vi "VisionDriver.vi"() -> (0 "horizontal":T2, 1 "vertical":T1)   [LabVIEW 2015]
uses:
  Robot Vision/horizontal.ctl
  Robot Vision/vertical.ctl
  Robot Vision/Robot Global Data.vi
panel:
  out "Distance (ft)":dbl
  out "Up":bool
  out "Down":bool
  out "Straight":bool
  out "Right":bool=TRUE
  out "Left":bool=TRUE
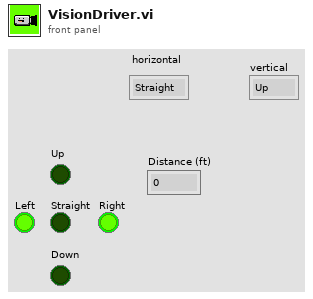
[diagram p1: front panel]
types:
  T1 = typedef "vertical.ctl" = enum16{"Up", "Down", "Straight"}
  T2 = typedef "horizontal.ctl" = enum16{"Straight", "Right", "Left"}
  T3 = cluster{"Distance (ft)":dbl, "Center":cluster{dbl, dbl}, "Normalized Rect":cluster{"Numeric":dbl, "Numeric 2":dbl, "Numeric 3":dbl, "Numeric 5":dbl}}[]
  T4 = cluster{"Distance (ft)":dbl, "Center":cluster{dbl, dbl}, "Normalized Rect":cluster{"Numeric":dbl, "Numeric 2":dbl, "Numeric 3":dbl, "Numeric 5":dbl}}
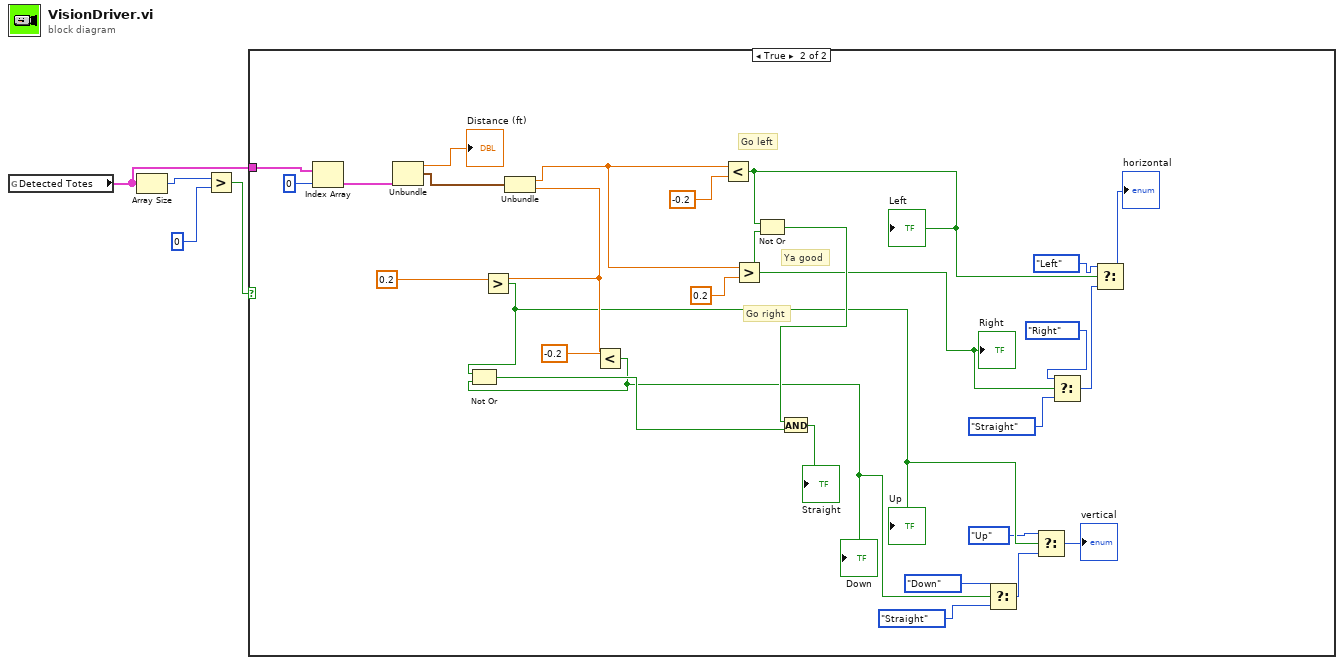
[diagram p0: block diagram]
diagram:
  n1 = global read "Robot Global Data.vi" "Detected Totes"() -> (w1:T3)
  n2 = Array Size(array=w1) -> (size(s)=w4:i32)
  n3 = Greater?(x=w4, y=0) -> (0:w2:bool)
  n4 = case shown="True" w2 {
    tunnel: w1 -> [_ w30]
    frame False {
    }
    frame True {
      # "Ya good"
      # "Go right"
      # "Go left"
      n5 = Index Array(array=w30, index=0) -> (element=w32:T4)
      n6 = Unbundle(w32) -> ("Distance (ft)"=→"Distance (ft)":dbl, "Center"=w29:cluster{dbl, dbl})  [unwired: 1 out]
      n7 = Unbundle(w29) -> (w28:dbl, w23:dbl)
      n8 = Greater?(x=w23, y=0.2 ("x")) -> (0:w11:bool)
      "Up" <- w11
      n9 = Less?(x=w23, y=-0.2 ("x")) -> (x < y?=w7:bool)
      "Down" <- w7
      n10 = Not Or(1:w7, 2:w11) -> (0:w20:bool)
      n11 = Less?(x=w28, y=-0.2) -> (x < y?=w18:bool)
      "Left" <- w18
      n12 = Greater?(x=w28, y=0.2) -> (0:w16:bool)
      "Right" <- w16
      n13 = Not Or(1:w16, 2:w18) -> (0:w21:bool)
      n14 = And(x=w21, y=w20) -> (x .and. y?=→"Straight":bool)
      n15 = Select(t=vertical."Down" ("vertical"), s=w7, f=vertical."Straight" ("vertical")) -> (s? t:f=w8:T1)
      n16 = Select(t=vertical."Up" ("vertical"), s=w11, f=w8) -> (s? t:f=→"vertical":T1)
      n17 = Select(t=horizontal."Right" ("horizontal"), s=w16, f=horizontal."Straight" ("horizontal")) -> (s? t:f=w17:T2)
      n18 = Select(t=horizontal."Left" ("horizontal"), s=w18, f=w17) -> (s? t:f=→"horizontal":T2)
    }
  }
